vi "Test Reading and Writing JSON Config.vi"() -> ()   [LabVIEW 2021]
uses:
  Source/Bool/conc_SharedVar_Bool.lvclass
  C:/Program Files (x86)/National Instruments/LabVIEW 2021/vi.lib/TSA/Abstract Data Classes/Abs_Types/Type/Abs_Type.lvclass
  <vilib>/TSA/Abstract Data Classes/Abs_Types/Boolean/Abs_Boolean.lvclass
  <vilib>/TSA/Abstract Data Classes/Abs_Types/Type/Abs_Type.lvclass/Abs_Type.ctl
  <vilib>/TSA/Abstract Data Classes/Abs_Types/Type/Properties/Write Name.vi
  <vilib>/TSA/Abstract Data Classes/Abs_Types/Type/Abs_Type.lvclass
panel:
  in  "Bool":bool
  out "Boolean":bool
  in  "stop":bool
  out "JSON":string
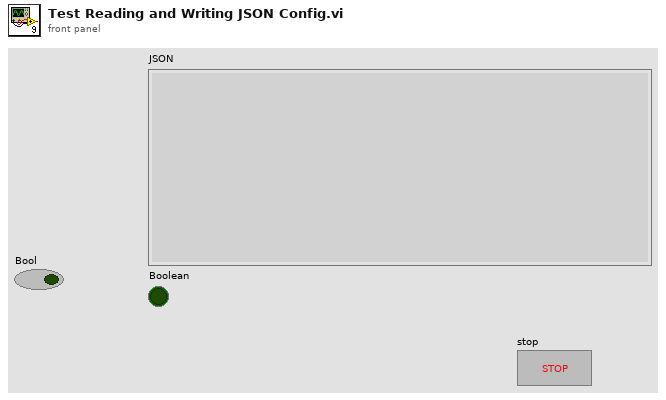
[diagram p1: front panel]
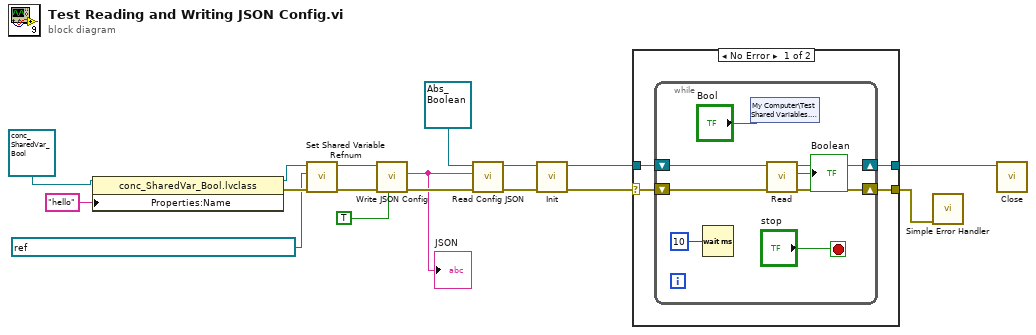
[diagram p0: block diagram]
diagram:
  n1 = property class="conc_SharedVar_Bool.lvclass"(reference=refnum<class "conc_SharedVar_Bool.lvclass"> refnum ("abs_SharedVar_Bool in"), "Properties:Name"="hello" ("Name")) -> (reference out=w5:refnum<class "conc_SharedVar_Bool.lvclass">, error out=w6:errorcluster)  [unwired: 1 in]
  n2 = call-dynamic "Set Shared Variable Refnum.vi"("error in (no error)"=w6, "shared variable refnum"=refnum<k21> "ni.var.psp://localhost/Test Shared Variables/Bool", "abs_SharedVar_Bool in"=w5) -> ("error out"=w2:errorcluster, "abs_SharedVar_Bool out"=w3:refnum<class "conc_SharedVar_Bool.lvclass">)  [unwired: 7 in]
  n3 = call-dynamic "Write JSON Config.vi"("Pretty Print?"=TRUE, "error in (no error)"=w2, "abs_SharedVar_Bool in"=w3) -> ("error out"=w10:errorcluster, "JSON"=w7:string)  [unwired: 6 in, 1 out]
  "JSON" <- w7
  n4 = call <vilib>:"Read Config JSON.vi"("error in (no error)"=w10, "JSON Config"=w7, "Abs_Type in"=refnum<class "Abs_Boolean.lvclass"> refnum ("Abs_Boolean.lvclass")) -> ("error out"=w11:errorcluster, "Abs_Type out"=w8:refnum<class "Abs_Boolean.lvclass">)  [unwired: 7 in]
  n5 = call-dynamic "Init.vi"("error in (no error)"=w11, "Data in"=w8) -> ("error out"=w13:errorcluster, "Data out"=w14:refnum<class "Abs_Boolean.lvclass">)  [unwired: 8 in]
  n6 = case shown="No Error" w13 {
    selector: w13 -> [w20 w30]
    tunnel: w14 -> [w21 w31]
    tunnel: [w19 w31] -> w12
    tunnel: [w18 w30] -> w1
    frame No Error {
      n7 = while {
        shift-right: [w27] -> w19
        shift-left: w21 -> [w29]
        shift-right: [w26] -> w18
        shift-left: w20 -> [w28]
        stop <- "stop" stop-if-true
        n8 = Wait (ms)(milliseconds to wait=u32 10) -> ()  [unwired: 1 out]
        n9 = shared-variable "My Computer\\Test Shared Variables.lvlib\\Bool"("Bool") -> ()  [unwired: 1 in, 1 out]
        n10 = call-dynamic "Read.vi"("error in (no error)"=w28, "Boolean in"=w29) -> ("error out"=w26:errorcluster, "Boolean"=→"Boolean":bool, "Boolean out"=w27:refnum<class "Abs_Boolean.lvclass">)  [unwired: 7 in]
      }
    }
    frame Error {
    }
  }
  n11 = call <vilib>:"Simple Error Handler.vi"("error in (no error)"=w1) -> ()  [unwired: 4 in, 5 out]
  n12 = call-dynamic "Close.vi"("Data in"=w12) -> ()  [unwired: 9 in, 2 out]
